vi "kinectRead [ColorFrame].vi"(8 "error in (no error)":errorcluster, 11 "KinectSensor References in":T1) -> (0 "error out":errorcluster, 2 "frameData":u8[](array[numeric]), 3 "KinectSensor References out":T1)   [LabVIEW 2014]
uses:
  controls/KinectSensor References.ctl
  Microsoft.Kinect
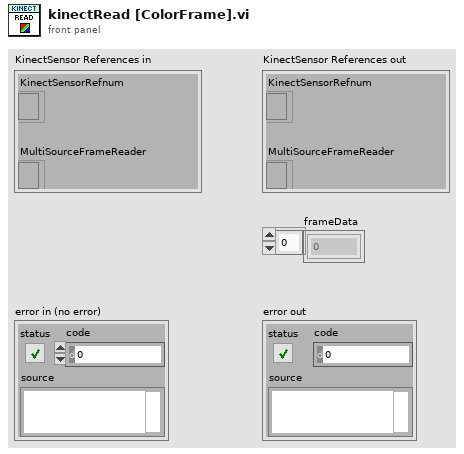
[diagram p1: front panel]
types:
  T1 = typedef "KinectSensor References.ctl" = cluster{"KinectSensorRefnum":refnum<k24>, "MultiSourceFrameReader":refnum<k24>}
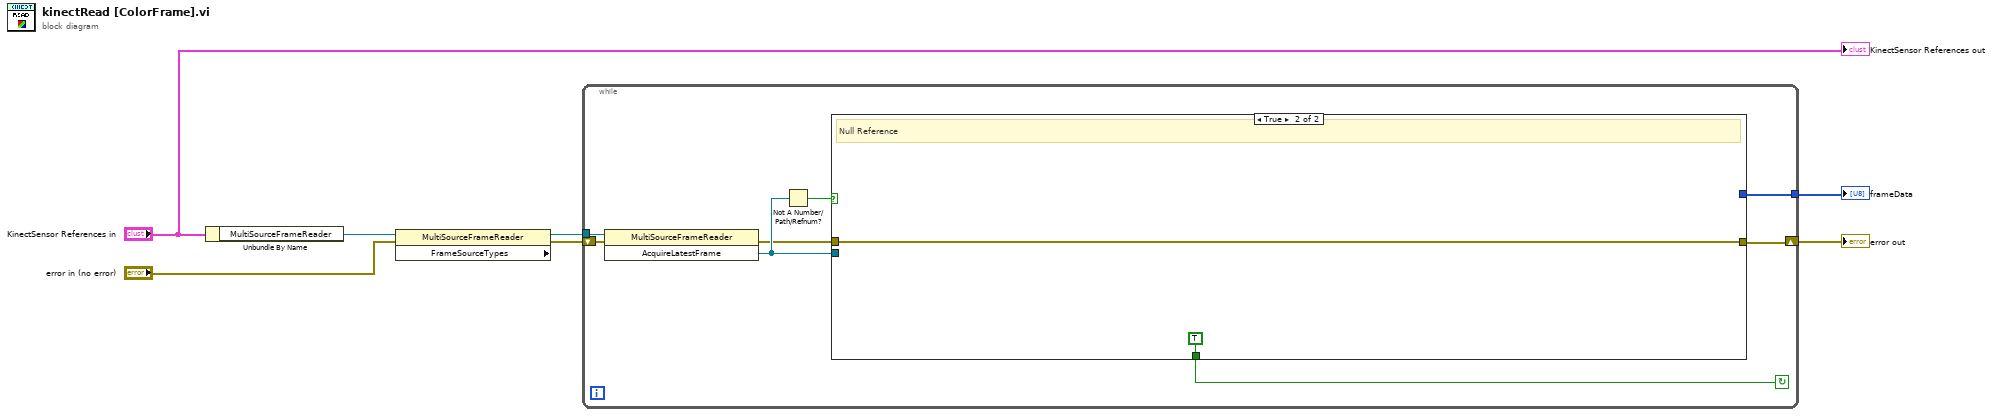
[diagram p0: block diagram]
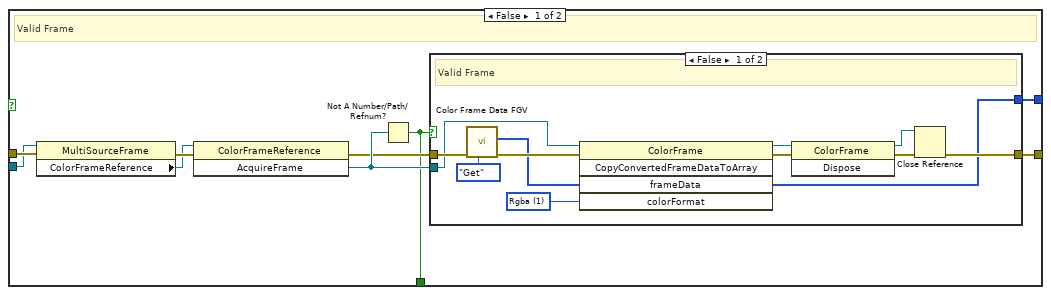
[diagram p2: hidden frame]
diagram:
  n1 = Unbundle By Name("KinectSensor References in") -> ("MultiSourceFrameReader"=w5:refnum<k24>)
  n2 = property class="MultiSourceFrameReader" props=["FrameSourceTypes"](reference=w5, error in="error in (no error)") -> (reference out=w7:refnum<k24>, error out=w6:errorcluster)  [unwired: 1 out]
  n3 = while {
    tunnel: w7 -> [w15]
    shift-right: [w10] -> w2
    shift-left: w6 -> [w14]
    tunnel: [w8] -> w1
    stop <- w9 continue-if-true
    n4 = invoke class="MultiSourceFrameReader" method="AcquireLatestFrame"(reference=w15, error in=w14) -> (error out=w12:errorcluster, "AcquireLatestFrame"=w13:refnum<k24>)  [unwired: 1 in, 1 out]
    n5 = Not A Number/Path/Refnum?(number/path/refnum=w13) -> (NaN/Path/Refnum?=w11:bool)
    n6 = case shown="True" w11 {
      tunnel: w12 -> [w21 w38]
      tunnel: w13 -> [w18 _]
      tunnel: [w20 w38] -> w10
      tunnel: [w19 TRUE] -> w9
      tunnel: [w16 _] -> w8
      frame False {
        # "Valid Frame"
        n7 = property class="MultiSourceFrame"(reference=w18, error in=w21) -> (error out=w22:errorcluster, "ColorFrameReference"=w17:refnum<k24>)  [unwired: 1 out]
        n8 = invoke class="ColorFrameReference" method="AcquireFrame"(reference=w17, error in=w22) -> (error out=w23:errorcluster, "AcquireFrame"=w24:refnum<k24>)  [unwired: 1 in, 1 out]
        n9 = Not A Number/Path/Refnum?(number/path/refnum=w24) -> (NaN/Path/Refnum?=w19:bool)
        n10 = case shown="False" w19 {
          tunnel: w23 -> [w28 w37]
          tunnel: w24 -> [w27 _]
          tunnel: [w26 w37] -> w20
          tunnel: [w25 _] -> w16
          frame False {
            w29 = 1 items=["None", "Rgba", "Yuv", "Bgra", "Bayer", "Yuy2"] ("colorFormat")
            # "Valid Frame"
            n11 = call "Color Frame Data FGV.vi"("Command"=enum16{"Get", "Initialize"}."Get", "error in (no error)"=w28) -> ("error out"=w36:errorcluster, "Byte Array"=w31:u8[])  [unwired: 8 in]
            n12 = invoke class="ColorFrame" method="CopyConvertedFrameDataToArray"(reference=w27, error in=w36, "frameData"=w31, "colorFormat"=w29) -> (reference out=w32:refnum<k24>, error out=w33:errorcluster, "frameData"=w25:u8[])  [unwired: 1 in, 2 out]
            n13 = invoke class="ColorFrame" method="Dispose"(reference=w32, error in=w33) -> (reference out=w35:refnum<k24>, error out=w34:errorcluster)  [unwired: 1 in, 1 out]
            n14 = Close Reference(reference=w35, error in (no error)=w34) -> (error out=w26:errorcluster)
          }
          frame True {
            # "Null Reference"
          }
        }
      }
      frame True {
        # "Null Reference"
      }
    }
  }
  "error out" <- w2
  "frameData" <- w1
  "KinectSensor References out" <- "KinectSensor References in"
